vi "macro_SimpleMotorFF_Ka_AutoTune.vi"   [LabVIEW 2019, in "Trajectory_Library.lvlib"]
uses:
  Trajectory_Library.lvlib
types:
  T1 = typedef "Trajectory_Library.lvlib/SIMPLE_MOTOR_FF_KA_TUNE_PARAMS.ctl" = cluster{"Max SP":dbl, "Min Eval SP":dbl, "Max Eval SP":dbl, "Ramp Rate":dbl}
  T2 = typedef "Trajectory_Library.lvlib/SIMPLE_MOTOR_FF.ctl" = cluster{"Ks":dbl, "Kv":dbl, "Ka":dbl, "KnInv":dbl}
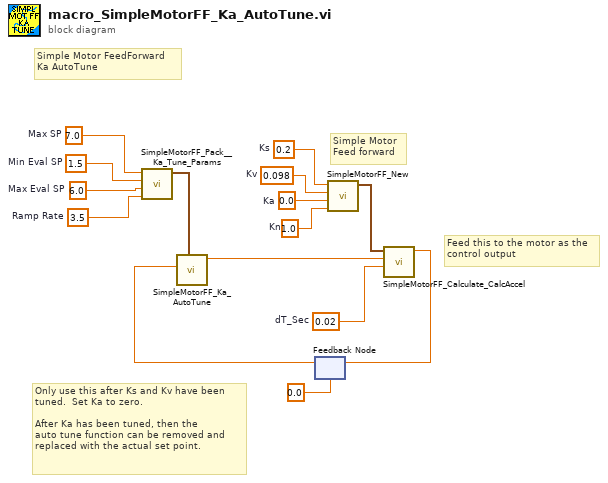
[diagram p0: block diagram]
diagram:
  w5 = 1.0  # Kn
  w6 = 0.02  # dT_Sec
  w8 = 0.2  # Ks
  w9 = 0.098  # Kv
  w10 = 0.0  # Ka
  w11 = 7.0  # Max SP
  w12 = 1.5  # Min Eval SP
  w13 = 6.0  # Max Eval SP
  w14 = 3.5  # Ramp Rate
  # "Only use this after Ks and Kv have been\ntuned.  Set Ka to zero.\n\nAfter Ka has been tuned, then the \nauto tune function can be removed and\nreplaced with the actual set point."
  # "Feed this to the motor as the\ncontrol output"
  # "Simple Motor\nFeed forward"
  # "Simple Motor FeedForward\nKa AutoTune"
  n1 = call "SimpleMotorFF_Pack__Ka_Tune_Params.vi"("Ramp Rate"=w14, "Max Eval SP"=w13, "Min Eval SP"=w12, "Max SP"=w11) -> ("Packed Params"=w15:T1)  [unwired: 7 in]
  n2 = feedback #1(0.0 ("FeedForward")) -> (w2:dbl)
  n3 = call "SimpleMotorFF_Ka_AutoTune.vi"("SimpleMotorFeedforward_KaTune_Pack"=w15, "CO Control Output"=w2) -> ("SP Setpoint"=w4:dbl)  [unwired: 3 in, 6 out]
  n4 = call "SimpleMotorFF_New.vi"("Kn"=w5, "Ka"=w10, "Kv"=w9, "Ks"=w8) -> ("SIMPLE_MOTOR_FF"=w7:T2)  [unwired: 7 in]
  n5 = call "SimpleMotorFF_Calculate_CalcAccel.vi"("dT_Sec"=w6, "VelSp"=w4, "SIMPLE_MOTOR_FF"=w7) -> ("FeedForward"=w3:dbl)  [unwired: 8 in]
  n6 = feedback-in #1(w3) -> ()
